vi "si_read_temperature.vi"() -> (1 "Read Temperature":dbl)   [LabVIEW 2011]
doc: "This VI reads the the thermal head through the controller.\n\n\nOutputs:\n1. Read Temperature : The actual temperature read by the controller."
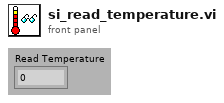
[diagram p1: front panel]
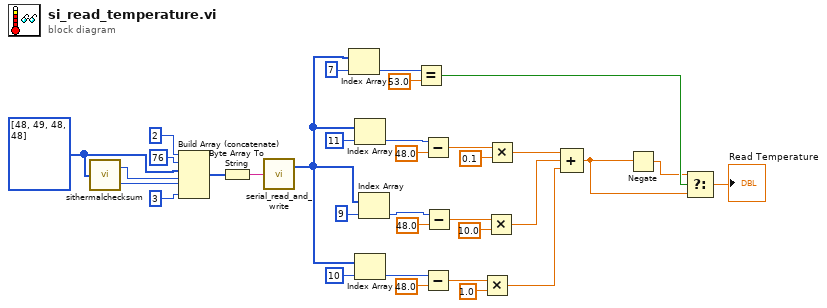
[diagram p0: block diagram]
diagram:
  w13 = i16[] [48, 49, 48, 48] ("Array")
  n1 = call "sithermalchecksum.vi"("Array"=w13) -> ("Lower Checksum"=w11:u8, "Upper Checksum"=w12:u8)
  n2 = Build Array (concatenate)(2, 76, w13, w12, w11, 3) -> (w10:i32[])
  n3 = Byte Array To String(unsigned byte array=w10) -> (string=w34:string)
  n4 = call "serial_read_and_write.vi"("write buffer"=w34) -> ("unsigned byte array"=w5:u8[])  [unwired: 1 in]
  n5 = Index Array(array=w5, index=7) -> (element=w9:u8)
  n6 = Index Array(array=w5, index=11) -> (element=w8:u8)
  n7 = Index Array(array=w5, index=10) -> (element=w6:u8)
  n8 = Index Array(array=w5, index=9) -> (element=w7:u8)
  n9 = Equal?(x=w9, y=53.0) -> (x = y?=w4:bool)
  n10 = Subtract(x=w8, y=48.0) -> (x-y=w32:dbl)
  n11 = Subtract(x=w6, y=48.0) -> (x-y=w28:dbl)
  n12 = Subtract(x=w7, y=48.0) -> (x-y=w24:dbl)
  n13 = Multiply(x=w28, y=1.0) -> (x*y=w19:dbl)
  n14 = Multiply(x=w24, y=10.0) -> (x*y=w20:dbl)
  n15 = Multiply(x=w32, y=0.1) -> (x*y=w21:dbl)
  n16 = Compound Arithmetic op=ADD(w21, w20, w19) -> (w2:dbl)
  n17 = Negate(x=w2) -> (-x=w3:dbl)
  n18 = Select(t=w3, s=w4, f=w2) -> (s? t:f=→"Read Temperature":dbl)
